vi "Jump to CSM State.vi"(6 "Config Path (\"\" For Lvcsm File)":path, 7 "Application Reference (Local)":refnum<vi>, 8 "error in (no error)":errorcluster, 9 "Type":enum16{"CSM", "CSM-VI"}(ring), 10 "State":string, 11 "Name":string) -> (0 "error out":errorcluster)   [LabVIEW 2017, in "CSM-Helper API with lvcsm Support.lvlib"]
uses:
  CSM-Helper API with lvcsm Support.lvlib
  4183b97d-67e9-48d0-9013-287ea012034b.vi
  901ca4ca-129f-45f5-aaf1-2c7f5df1094f.vi
  API/Destroy.vi
  API/Set Visible Case Frame.vi
  API/Open Block Diagram.vi
  API/Create From VI Reference.vi
  lvcsmFile/_Array of VData to VCluster.vi
  <vilib>/Utility/config.llb/Close Config Data.vi
  <vilib>/Utility/config.llb/Read Key.vi
  <vilib>/Utility/config.llb/Read Key (Double).vi
  <vilib>/Utility/config.llb/Read Key (I32).vi
  lvcsmFile/lvcsm String to Path.vi
  <vilib>/Utility/config.llb/Read Key (String).vi
  lvcsmFile/Path to lvcsm String.vi
  <vilib>/Utility/config.llb/Get Key Names.vi
  <vilib>/Utility/Data Type/Get Type Information.vi
  <vilib>/Utility/Data Type/Get Array Information.vi
  <vilib>/Utility/config.llb/Read Key (Boolean).vi
  <vilib>/Utility/config.llb/Open Config Data.vi
  lvcsmFile/lvcsm File Path.vi
  CSM-Helper.lvclass
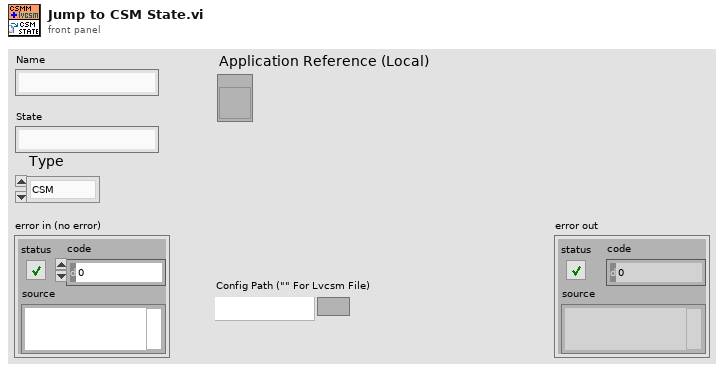
[diagram p1: front panel]
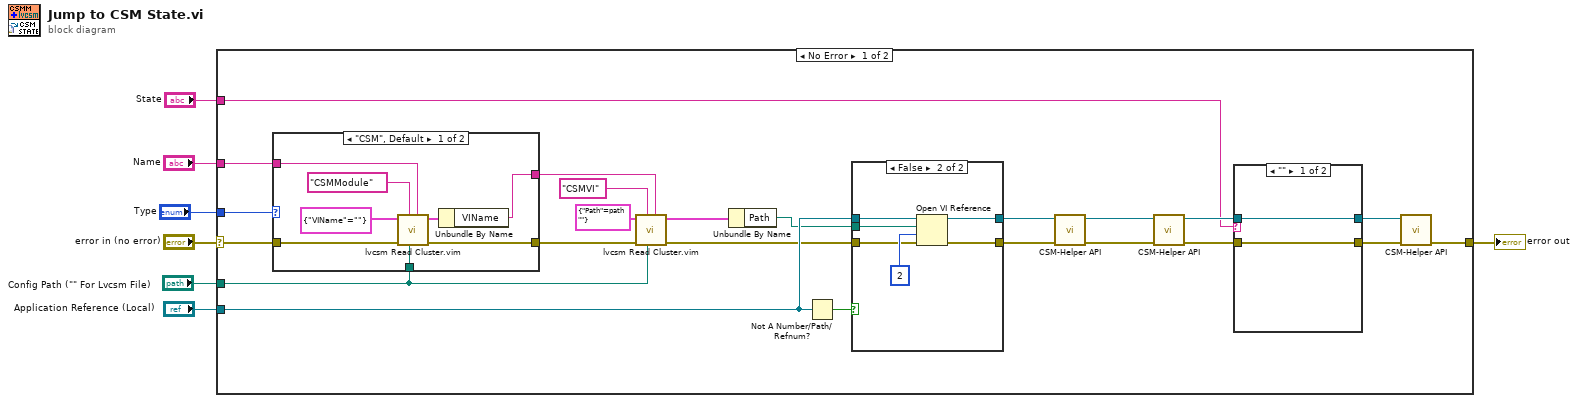
[diagram p0: block diagram]
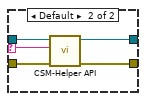
[diagram p2: hidden frame]
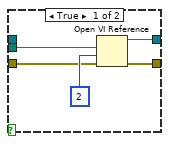
[diagram p4: hidden frame]
diagram:
  n1 = case shown="No Error" "error in (no error)" {
    selector: "error in (no error)" -> [w30 w59]
    tunnel: [w19 w59] -> w7
    tunnel: "Name" -> [w29 _]
    tunnel: "Config Path (\"\" For Lvcsm File)" -> [w10 _]
    tunnel: "State" -> [w22 _]
    tunnel: "Application Reference (Local)" -> [w18 _]
    tunnel: "Type" -> [w8 _]
    frame No Error {
      n2 = case shown="\"CSM\", Default" w8 {
        tunnel: w30 -> [w45 w47]
        tunnel: w29 -> [w43 w46]
        tunnel: [w40 w46] -> w13
        tunnel: [w39 w47] -> w11
        tunnel: w10 -> [w38 _]
        frame "CSM", Default {
          n3 = call "lvcsm Read Cluster.vim"("Sub-section (\"\")"=w43, "Config Path"=w38, "Section"="CSMModule", "Error In"=w45, "Default Prototype"=cluster{"VIName":string} {"VIName"=""}) -> ("error out"=w39:errorcluster, "Cluster (Dup)"=w41:cluster{"VIName":string})  [unwired: 5 in]
          n4 = Unbundle By Name(w41) -> ("VIName"=w40:string)
        }
        frame "CSM-VI" {
        }
      }
      n5 = call "lvcsm Read Cluster.vim"("Sub-section (\"\")"=w13, "Config Path"=w10, "Section"="CSMVI", "Error In"=w11, "Default Prototype"=cluster{"Path":path} {"Path"=path ""}) -> ("error out"=w12:errorcluster, "Cluster (Dup)"=w16:cluster{"Path":path})  [unwired: 5 in]
      n6 = Unbundle By Name(w16) -> ("Path"=w9:path)
      n7 = Not A Number/Path/Refnum?(number/path/refnum=w18) -> (NaN/Path/Refnum?=w17:bool)
      n8 = case shown="False" w17 {
        tunnel: [w52 w58] -> w28
        tunnel: [w51 w57] -> w27
        tunnel: w12 -> [w49 w55]
        tunnel: w18 -> [_ w54]
        tunnel: w9 -> [w48 w53]
        frame True {
          n9 = Open VI Reference(vi path=w48, options=2, error in (no error)=w49) -> (vi reference=w51:refnum<vi>, error out=w52:errorcluster)  [unwired: 3 in]
        }
        frame False {
          n10 = Open VI Reference(application reference (local)=w54, vi path=w53, options=2, error in (no error)=w55) -> (vi reference=w57:refnum<vi>, error out=w58:errorcluster)  [unwired: 2 in]
        }
      }
      n11 = call-poly "CSM-Helper API.vi"("error in (no error)"=w28, "VI"=w27) -> ("error out"=w26:errorcluster, "CSM-Helper.lvclass"=w25:refnum<class "CSM-Helper.lvclass">)  [unwired: 8 in]
      n12 = call-poly "CSM-Helper API.vi"("error in (no error)"=w26, "CSM-Helper in"=w25) -> ("error out"=w24:errorcluster, "CSM-Helper out"=w23:refnum<class "CSM-Helper.lvclass">)  [unwired: 8 in]
      n13 = case shown="\"\"" w22 {
        selector: w22 -> [_ w35]
        tunnel: w24 -> [w31 w37]
        tunnel: w23 -> [w32 w36]
        tunnel: [w31 w34] -> w21
        tunnel: [w32 w33] -> w20
        frame "" {
        }
        frame Default {
          n14 = call-poly "CSM-Helper API.vi"("error in (no error)"=w37, "element"=w35, "CSM-Helper in"=w36) -> ("error out"=w34:errorcluster, "CSM-Helper out"=w33:refnum<class "CSM-Helper.lvclass">)  [unwired: 7 in]
        }
      }
      n15 = call-poly "CSM-Helper API.vi"("error in (no error)"=w21, "CSM-Helper in"=w20) -> ("error out"=w19:errorcluster)  [unwired: 8 in, 1 out]
    }
    frame Error {
    }
  }
  "error out" <- w7
